vi "Copy VI and disconnect it from library.vi"(8 "error in (no error)":errorcluster, 10 "VI Target Path":path, 11 "VI Source Path":path) -> (0 "error out":errorcluster)   [LabVIEW 2015]
doc: "Copy an existing VI from the source path to the destination path and disconnect it from the owning library."
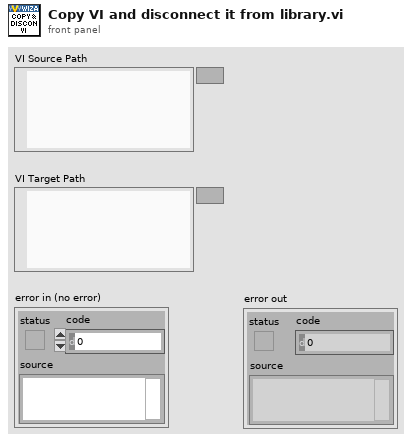
[diagram p1: front panel]
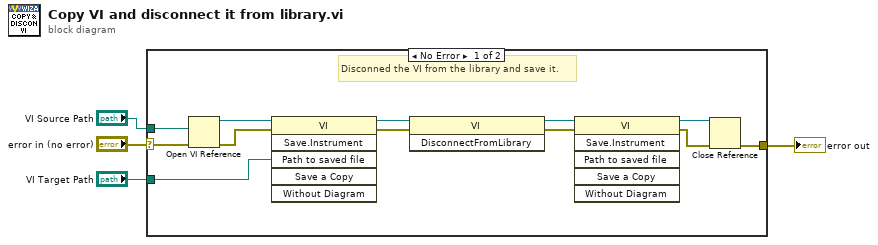
[diagram p0: block diagram]
diagram:
  n1 = case shown="No Error" "error in (no error)" {
    selector: "error in (no error)" -> [w16 w17]
    tunnel: [w15 w17] -> w4
    tunnel: "VI Source Path" -> [w14 _]
    tunnel: "VI Target Path" -> [w13 _]
    frame No Error {
      # "Disconned the VI from the library and save it."
      n2 = Open VI Reference(vi path=w14, error in (no error)=w16) -> (vi reference=w12:refnum<vi>, error out=w10:errorcluster)  [unwired: 4 in]
      n3 = invoke class="VI" method="Save.Instrument"(reference=w12, error in=w10, "Path to saved file"=w13) -> (reference out=w11:refnum<vi>, error out=w9:errorcluster)  [unwired: 3 in, 4 out]
      n4 = invoke class="VI" method="DisconnectFromLibrary"(reference=w11, error in=w9) -> (reference out=w8:refnum<vi>, error out=w7:errorcluster)  [unwired: 1 in, 1 out]
      n5 = invoke class="VI" method="Save.Instrument"(reference=w8, error in=w7) -> (reference out=w6:refnum<vi>, error out=w5:errorcluster)  [unwired: 4 in, 4 out]
      n6 = Close Reference(reference=w6, error in (no error)=w5) -> (error out=w15:errorcluster)
    }
    frame Error {
      # "Output default values."
    }
  }
  "error out" <- w4
